vi "Element Init.vi"(7 "VolatusAPI":refnum<class "VolatusAPI.lvclass">, 8 "error in (no error)":errorcluster, 10 "JSON":string, 11 "NumericIndicator in":refnum<class "NumericIndicator.lvclass">) -> (0 "error out":errorcluster, 3 "NumericIndicator out":refnum<class "NumericIndicator.lvclass">)   [LabVIEW 2020, in "VolatusGUIElements.lvlib" / "NumericIndicator.lvclass"]
uses:
  NumericIndicator.lvclass
  Volatus/VolatusAPI/VolatusAPI.lvclass
  JSON.ctl
  lv-vecto/Vecto/Group DBL/Group DBL.lvclass
  C:/dev/lv20CE/relink/lv-vecto/Vecto/Group/Group.lvclass
  NumericIndicator.lvclass/NumericIndicator.ctl
  bc1d0ba6-3274-416f-84ea-d61b916d66ff.vi
  <vilib>/JDP Science/JSONtext/JSON text to Variant.vi
  <vilib>/JDP Science/JSONtext/LVClass Serializer/JSONtext LVClass Serializer.lvclass
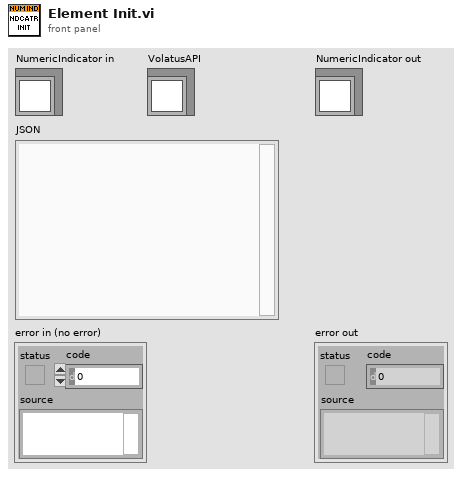
[diagram p1: front panel]
types:
  T1 = typedef "VolatusGUIElements.lvlib/NumericIndicator.lvclass/JSON.ctl" = cluster{"Channel":string}
  T2 = typedef "VectoConfig.lvlib/Channel Info.ctl" = cluster{"Name":string, "Group":string, "Owning Node":string, "Owning Task":string, "Resource":string}
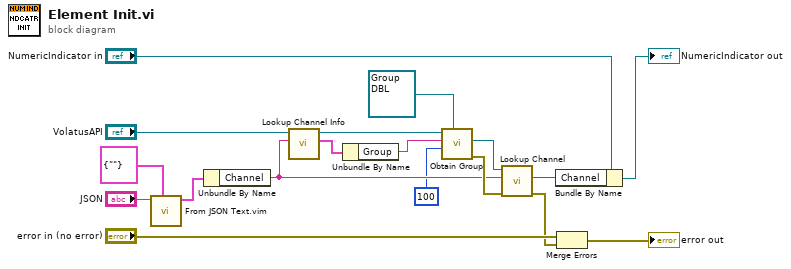
[diagram p0: block diagram]
diagram:
  n1 = call "From JSON Text.vim"("Data Type and Default Value"=T1 {"Channel"=""} ("JSON"), "JSON"="JSON") -> ("Data out"=w13:T1)  [unwired: 8 in, 1 out]
  n2 = Unbundle By Name(w13) -> ("Channel"=w4:string)
  n3 = call "Lookup Channel Info.vi"("Channel Name"=w4, "VolatusAPI in"="VolatusAPI") -> ("Channel Info"=w3:T2, "VolatusAPI out"=w5:refnum<class "VolatusAPI.lvclass">)  [unwired: 6 in, 2 out]
  n4 = Unbundle By Name(w3) -> ("Group"=w2:string)
  n5 = call "Obtain Group.vi"("Group Type (Abstract)"=refnum<class "Group DBL.lvclass"> refnum ("Group in"), "Timeout ms (5000)"=u32 100, "Group Name"=w2, "VolatusAPI in"=w5) -> ("error out"=w18:errorcluster, "Group"=w6:refnum<class "Group DBL.lvclass">)  [unwired: 5 in, 1 out]
  n6 = call "Lookup Channel.vi"("error in (no error)"=w18, "Channel Name"=w4, "Group in"=w6) -> ("error out"=w9:errorcluster, "Channel"=w11:refnum<class "Channel DBL.lvclass">)  [unwired: 6 in, 1 out]
  n7 = Bundle By Name(cluster="NumericIndicator in", "Channel"=w11) -> (→"NumericIndicator out":refnum<class "NumericIndicator.lvclass">)
  n8 = Merge Errors("error in (no error)", w9) -> (→"error out":errorcluster)
